vi "SECoP_dataFromJSON.vi"(8 "error in (no error)":errorcluster, 9 "hint: SECoP_dataPtr":T1 {"ptr64" format="%.0x"; "ptr32" format="%.0x"}, 10 "JSON":string, 11 "DLL path (in)":T2) -> (0 "error out":errorcluster, 2 "SECoP_dataPtr (out)":T1 {"ptr64" format="%.0x"; "ptr32" format="%.0x"}, 3 "DLL path (out)":T2)   [LabVIEW 2023, in "SECoP.lvlib"]
doc: "Call <b>\"SECoP_dataFromJSON.vi\"</b> to convert a JSON value string to internal SECoP_dataPtr with an optional hint. A new value is created, free resources after use with <b>\"SECoP_dataDestroy.vi\"</b>.\n\n<b>DLL path</b> input and output of cluster from \"SECoP-Initialize.vi\"\n<b>SECoP_dataPtr</b> data to access\n<b>Position</b> points to a virtual flattened entry of the data type\n<b>struct_name</b> name of the requested struct item\n<b>index</b> found position of the requested struct item for direct access with <b>\"SECoP_data*.vi\"</b>"
uses:
  SECoP.lvlib
  SECoP-libraries.ctl
  SECoP-data.ctl
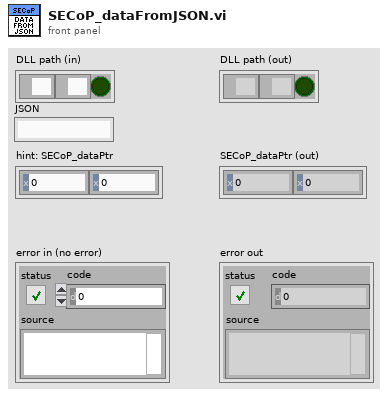
[diagram p1: front panel]
types:
  T1 = typedef "SECoP.lvlib/SECoP-data.ctl" = cluster{"ptr32":u32, "ptr64":u64}
  T2 = typedef "SECoP.lvlib/SECoP-libraries.ctl" = cluster{"serverDLL":path, "variantDLL":path, "cleanup_mode":bool}
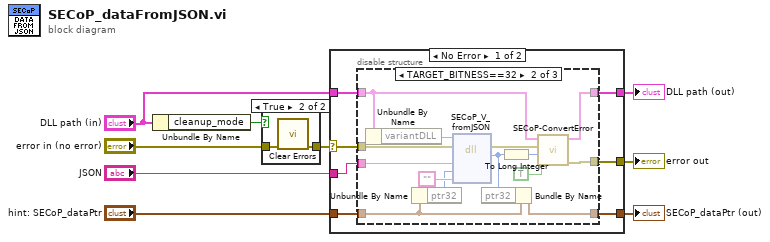
[diagram p0: block diagram]
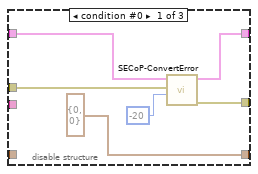
[diagram p3: hidden frame]
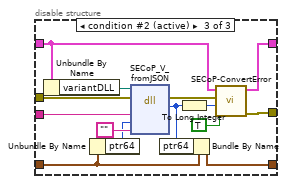
[diagram p4: hidden frame]
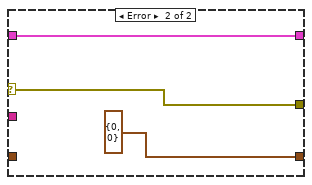
[diagram p5: hidden frame]
diagram:
  n1 = Unbundle By Name("DLL path (in)") -> ("cleanup_mode"=w7:bool)
  n2 = case shown="True" w7 {
    tunnel: "error in (no error)" -> [w10 w12]
    tunnel: [w10 w11] -> w5
    frame False {
    }
    frame True {
      n3 = call <vilib>:"Clear Errors.vi"("error in (no error)"=w12) -> ("error out"=w11:errorcluster)  [unwired: 5 in, 1 out]
    }
  }
  n4 = case shown="No Error" w5 {
    selector: w5 -> [w19 w55]
    tunnel: "DLL path (in)" -> [w18 w56]
    tunnel: [w16 w56] -> w9
    tunnel: [w17 w55] -> w8
    tunnel: "JSON" -> [w15 _]
    tunnel: "hint: SECoP_dataPtr" -> [w13 _]
    tunnel: [w14 T1 {"ptr32"=0, "ptr64"=0} ("hint: SECoP_dataPtr")] -> w1
    frame No Error {
      n5 = disable-structure shown="TARGET_BITNESS==32" {
        disable-tunnel: w19 -> [w23 w38 w52]
        disable-tunnel: w18 -> [w25 w27 w40]
        disable-tunnel: [w22 w32 w46] -> w17
        disable-tunnel: [w24 w33 w47] -> w16
        disable-tunnel: w15 -> [_ w37 w51]
        disable-tunnel: [T1 {"ptr32"=0, "ptr64"=0} ("hint: SECoP_dataPtr") w35 w49] -> w14
        disable-tunnel: w13 -> [_ w36 w50]
        frame condition #0 {
          n6 = call "SECoP-ConvertError.vi"("return code"=-20, "error in (no error)"=w23, "DLL path (in)"=w25) -> ("error out"=w22:errorcluster, "DLL path (out)"=w24:T2)  [unwired: 7 in]
        }
        frame condition #1 {
          n7 = Unbundle By Name(w27) -> ("variantDLL"=w26:path)
          n8 = Unbundle By Name(w36) -> ("ptr32"=w31:u32)
          n9 = dll-call lib="Z:/Praktische_Aufgaben/SECoP-LabVIEW2015/32bit/SECoP32.dll" fn="SECoP_V_fromJSON"(path in=w26, error in=w38, "JSON"=w37, "Hint"=w31, "Part"="") -> (error out=w34:errorcluster, "return type"=w30:u32)  [unwired: 4 in, 1 out]
          n10 = Bundle By Name(cluster=w36, "ptr32"=w30) -> (w35:T1)
          n11 = To Long Integer(number=w30) -> (32bit integer=w29:i32)
          n12 = call "SECoP-ConvertError.vi"("return is boolean"=TRUE, "return code"=w29, "error in (no error)"=w34, "DLL path (in)"=w27) -> ("error out"=w32:errorcluster, "DLL path (out)"=w33:T2)  [unwired: 6 in]
        }
        frame condition #2 (active) {
          n13 = Unbundle By Name(w40) -> ("variantDLL"=w41:path)
          n14 = Unbundle By Name(w50) -> ("ptr64"=w45:u64)
          n15 = dll-call lib="Z:/Praktische_Aufgaben/SECoP-LabVIEW2015/32bit/SECoP32.dll" fn="SECoP_V_fromJSON"(path in=w41, error in=w52, "JSON"=w51, "Hint"=w45, "Part"="") -> (error out=w48:errorcluster, "return type"=w44:u64)  [unwired: 4 in, 1 out]
          n16 = Bundle By Name(cluster=w50, "ptr64"=w44) -> (w49:T1)
          n17 = To Long Integer(number=w44) -> (32bit integer=w43:i32)
          n18 = call "SECoP-ConvertError.vi"("return is boolean"=TRUE, "return code"=w43, "error in (no error)"=w48, "DLL path (in)"=w40) -> ("error out"=w46:errorcluster, "DLL path (out)"=w47:T2)  [unwired: 6 in]
        }
      }
    }
    frame Error {
    }
  }
  "DLL path (out)" <- w9
  "error out" <- w8
  "SECoP_dataPtr (out)" <- w1
